vi "Tree Map to XML Recursive.vi"(7 "Indent":i32, 10 "Path Set":set{string}(c389), 11 "Tree Map In":T1) -> (3 "XML Lines":string[](array[string]), 4 "Path Invalid":bool)   [LabVIEW 2019, in "Tree Map.lvlib"]
doc: "<b>Author:</b> Piotr Kruczkowski <PrimaryKey>\n<b>License:</b> NewBSD\n\nCopyright (c) 2019, National Instruments\nAll rights reserved.\n\nRedistribution and use in source and binary forms, with or without\nmodification, are permitted provided that the following conditions are met:\n1. Redistributions of source code must retain the above copyright\n notice, this list of conditions and the following disclaimer.\n2. Redistributions in binary form must reproduce the above copyright\n notice, this list of conditions and the following disclaimer in the\n documentation and/or other materials provided with the distribution.\n3. Neither the name of National Instruments nor the\n names of its contributors may be used to endorse or promote products\n derived from this software without specific prior written permission.\n\nTHIS SOFTWARE IS PROVIDED BY National Instruments ''AS IS'' AND ANY\nEXPRESS OR IMPLIED WARRANTIES, INCLUDING, BUT NOT LIMITED TO, THE IMPLIED\nWARRANTIES OF MERCHANTABILITY AND FITNESS FOR A PARTICULAR PURPOSE ARE\nDISCLAIMED. IN NO EVENT SHALL National Instruments BE LIABLE FOR ANY\nDIRECT, INDIRECT, INCIDENTAL, SPECIAL, EXEMPLARY, OR CONSEQUENTIAL DAMAGES\n(INCLUDING, BUT NOT LIMITED TO, PROCUREMENT OF SUBSTITUTE GOODS OR SERVICES;\nLOSS OF USE, DATA, OR PROFITS; OR BUSINESS INTERRUPTION) HOWEVER CAUSED AND\nON ANY THEORY OF LIABILITY, WHETHER IN CONTRACT, STRICT LIABILITY, OR TORT\n(INCLUDING NEGLIGENCE OR OTHERWISE) ARISING IN ANY WAY OUT OF THE USE OF THIS\nSOFTWARE, EVEN IF ADVISED OF THE POSSIBILITY OF SUCH DAMAGE."
uses:
  Tree Map.lvlib
  Tree Map Data.ctl
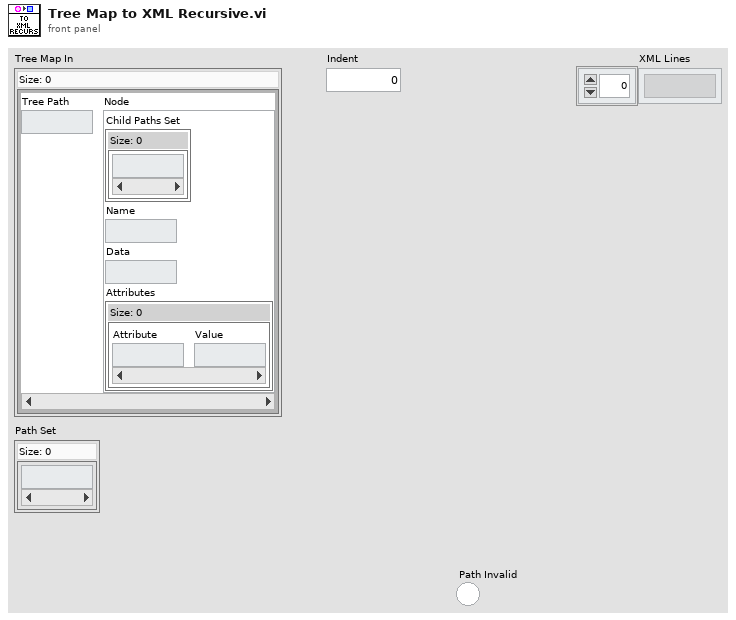
[diagram p1: front panel]
types:
  T1 = typedef "Tree Map.lvlib/Tree Map Data.ctl" = map{string, cluster{"Child Paths Set":set{string}, "Name":string, "Data":string, "Attributes":map{string, string}}}
  T2 = cluster{"Child Paths Set":set{string}, "Name":string, "Data":string, "Attributes":map{string, string}}
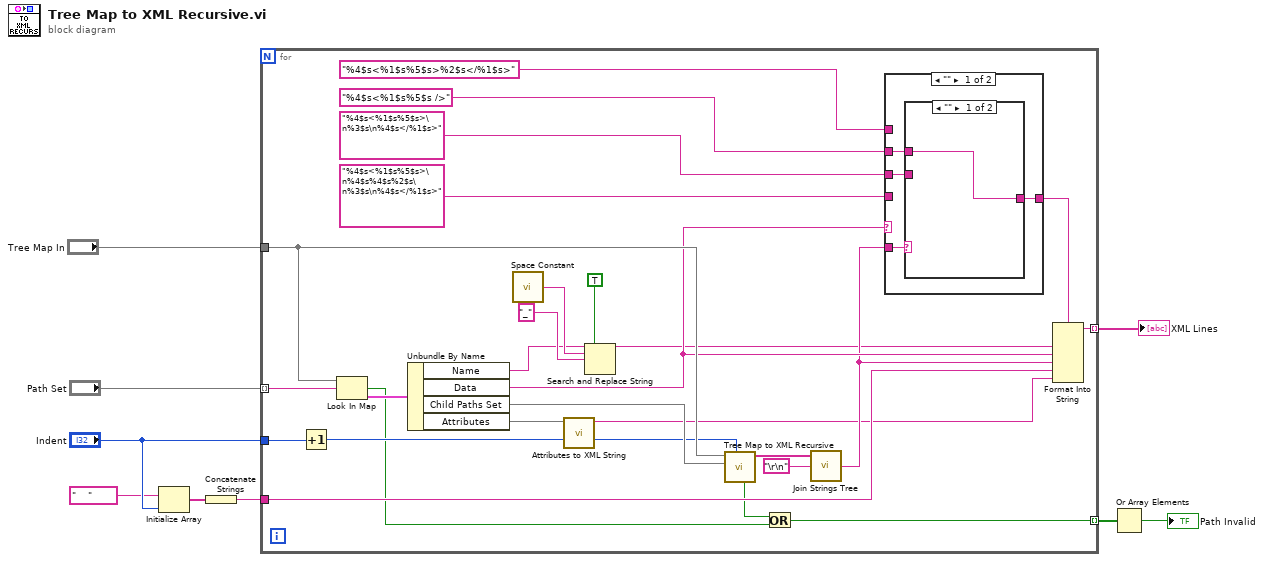
[diagram p0: block diagram]
diagram:
  n1 = Initialize Array("    ", "Indent") -> (w7:string[])
  n2 = Concatenate Strings(w7) -> (w8:string)
  n3 = for {
    tunnel: w8 -> [w30]
    tunnel: "Indent" -> [w36]
    tunnel: [w27] -> w5 mode=indexing
    tunnel: "Path Set" -> [w28] mode=indexing
    tunnel: "Tree Map In" -> [w33]
    tunnel: [w14] -> w3 mode=indexing
    n4 = Increment(x=w36) -> (x+1=w29:i32)
    n5 = Look In Map(map=w33, key=w28) -> (key not found?=w15:bool, value=w35:T2)  [unwired: 1 in]
    n6 = Unbundle By Name(w35) -> ("Name"=w10:string, "Data"=w26:string, "Child Paths Set"=w34:set{string}, "Attributes"=w12:map{string, string})
    n7 = call <vilib>:"Space Constant.vi"() -> ("String"=w20:string)
    n8 = call "Attributes to XML String.vi"("Attributes"=w12) -> ("XML String"=w11:string)  [unwired: 10 in]
    n9 = Search and Replace String(replace all?=TRUE ("replace all? (F)"), input string=w10, search string=w20, replace string="_") -> (result string=w17:string)  [unwired: 4 in, 3 out]
    n10 = call "Tree Map to XML Recursive.vi"("Indent"=w29, "Path Set"=w34, "Tree Map In"=w33) -> ("XML Lines"=w32:string[], "Path Invalid"=w16:bool)  [unwired: 7 in]
    n11 = Or(x=w16, y=w15) -> (x .or. y?=w14:bool)
    n12 = call "Join Strings Tree.vi"("Separator"="\r\n", "Strings In"=w32) -> ("String"=w25:string)  [unwired: 1 in]
    n13 = case shown="\"\"" w26 {
      tunnel: w25 -> [w40 w46]
      tunnel: "%4$s<%1$s%5$s>%2$s</%1$s>" ("format string") -> [_ w45]
      tunnel: "%4$s<%1$s%5$s>\n%4$s%4$s%2$s\n%3$s\n%4$s</%1$s>" ("format string") -> [_ w44]
      tunnel: [w39 w43] -> w24
      tunnel: "%4$s<%1$s%5$s>\n%3$s\n%4$s</%1$s>" ("format string") -> [w37 _]
      tunnel: "%4$s<%1$s%5$s />" ("format string") -> [w38 _]
      frame "" {
        n14 = case shown="\"\"" w40 {
          tunnel: [w41 w42] -> w39
          tunnel: w38 -> [w41 _]
          tunnel: w37 -> [_ w42]
          frame "" {
          }
          frame Default {
          }
        }
      }
      frame Default {
        n15 = case shown="\"\"" w46 {
          tunnel: w45 -> [w47 _]
          tunnel: w44 -> [_ w48]
          tunnel: [w47 w48] -> w43
          frame "" {
          }
          frame Default {
          }
        }
      }
    }
    n16 = Format Into String(format string=w24, w17, w26, w25, w30, w11) -> (resulting string=w27:string)  [unwired: 2 in, 1 out]
  }
  "XML Lines" <- w5
  n17 = Or Array Elements(Boolean array=w3) -> (logical OR=→"Path Invalid":bool)
